vi "ArcadeDrivePieceWise.vi"(8 "Cutoff":dbl=0.7 format="%#_13g", 9 "Direction":dbl format="%#_13g", 10 "Throttle":dbl format="%#_13g", 11 "Deadzone":dbl format="%#_13g") -> (1 "DriveRight":dbl, 2 "DriveLeft":dbl)   [LabVIEW 2013]
doc: "Based on the given throttle and direction, sets the left and right motor outputs. If direction is within deadzone, both motor outputs are zero. If direction is outside deadzone, the throttle is assigned to one side (depending on the sign of direction). The other side is scaled according to a piecewise function. If abs(direction) is less than cutoff, then the scale is linear. If abs(direction) is greater than cutoff, the scale is -1."
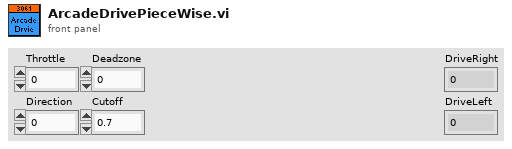
[diagram p1: front panel]
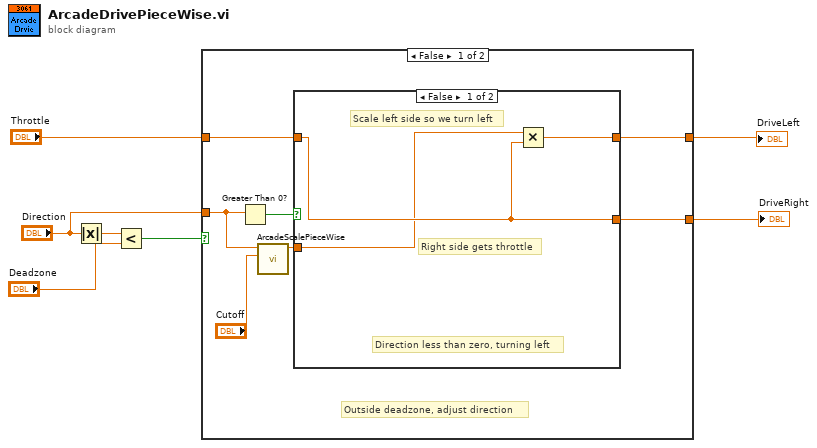
[diagram p0: block diagram]
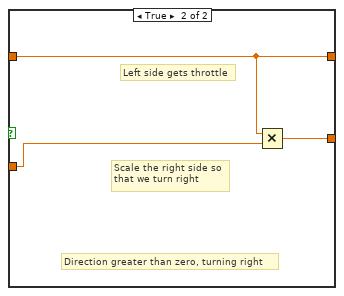
[diagram p2: hidden frame]
diagram:
  n1 = Absolute Value(x="Direction") -> (abs(x)=w6:dbl)
  n2 = Less?(x=w6, y="Deadzone") -> (x < y?=w4:bool)
  n3 = case shown="False" w4 {
    tunnel: "Throttle" -> [w14 w21]
    tunnel: [w12 w21] -> w2
    tunnel: [w11 w21] -> w3
    tunnel: "Direction" -> [w10 _]
    frame False {
      # "Outside deadzone, adjust direction"
      n4 = Greater Than 0?(x=w10) -> (x > 0?=w13:bool)
      n5 = call "ArcadeScalePieceWise.vi"("Cutoff"="Cutoff", "Direction"=w10) -> ("Scale"=w9:dbl)  [unwired: 9 in]
      n6 = case shown="False" w13 {
        tunnel: w14 -> [w17 w20]
        tunnel: [w15 w20] -> w12
        tunnel: w9 -> [w16 w19]
        tunnel: [w17 w18] -> w11
        frame False {
          # "Scale left side so we turn left"
          # "Right side gets throttle"
          # "Direction less than zero, turning left"
          n7 = Multiply(x=w16, y=w17) -> (x*y=w15:dbl)
        }
        frame True {
          # "Scale the right side so\nthat we turn right"
          # "Left side gets throttle"
          # "Direction greater than zero, turning right"
          n8 = Multiply(x=w20, y=w19) -> (x*y=w18:dbl)
        }
      }
    }
    frame True {
      # "Within deadzone, act like straight drive"
    }
  }
  "DriveRight" <- w3
  "DriveLeft" <- w2
